vi "Create Files.vi"(8 "error in (no error)":errorcluster, 11 "CubeLogger in":refnum<class "CubeLogger.lvclass">) -> (0 "error out":errorcluster, 2 "Canceled?":bool, 3 "CubeLogger out":refnum<class "CubeLogger.lvclass">)   [LabVIEW 2018, in "CubeLogger.lvclass"]
uses:
  CubeLogger.lvclass
  CubeLogger.lvclass/CubeLogger.ctl
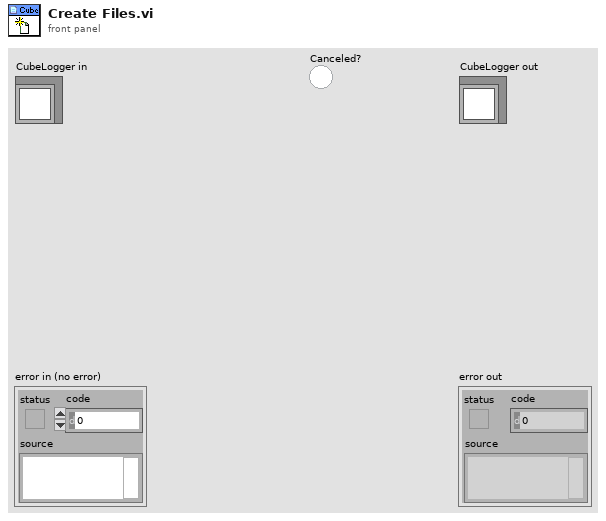
[diagram p1: front panel]
types:
  T1 = enum16{"open", "replace", "create", "open or create", "replace or create", "replace or create with confirmation"}
  T2 = typedef "CubeLogger.lvclass/Dataset.ctl" = cluster{"name":string, "path":string, "size":i32[], "type":enum16{"single", "double", "uint8", "uint16", "uint32", "uint64", "int8", "int16", "int32", "int64"}, "mfmt":string}
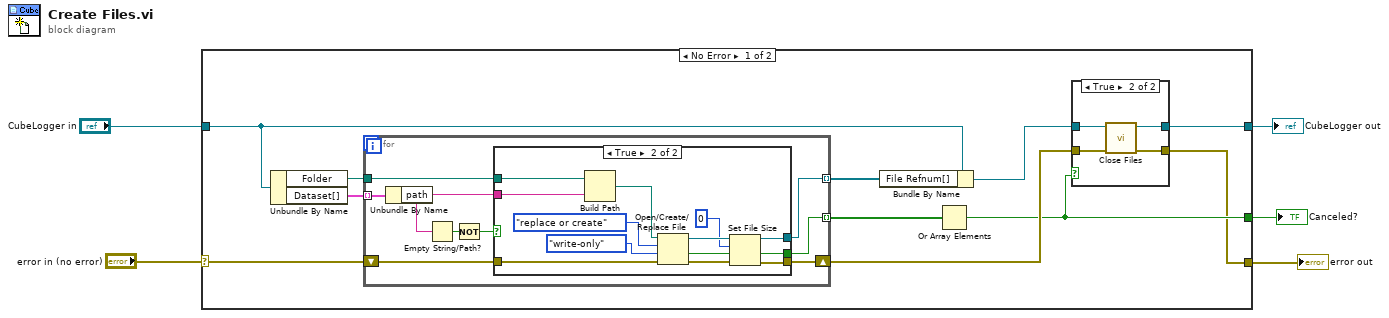
[diagram p0: block diagram]
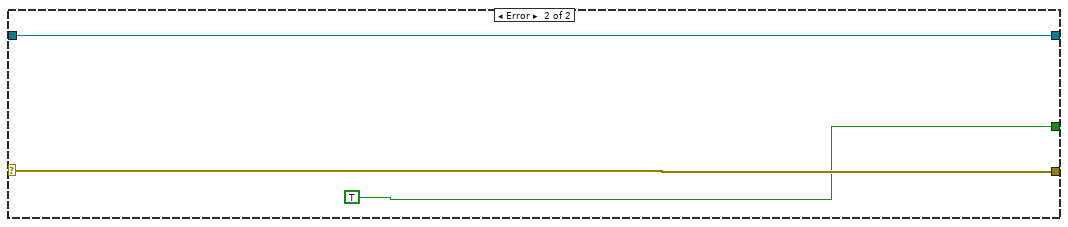
[diagram p4: hidden frame]
diagram:
  n1 = case shown="No Error" "error in (no error)" {
    selector: "error in (no error)" -> [w14 w47]
    tunnel: [w6 w47] -> w4
    tunnel: [w9 w46] -> w2
    tunnel: "CubeLogger in" -> [w12 w46]
    tunnel: [w7 TRUE] -> w1
    frame No Error {
      n2 = Unbundle By Name(w12) -> ("Folder"=w15:path, "Dataset[]"=w16:T2[])
      n3 = for {
        tunnel: w16 -> [w31] mode=indexing
        tunnel: w15 -> [w30]
        shift-right: [w28] -> w8
        shift-left: w14 -> [w29]
        tunnel: [w27] -> w13 mode=indexing
        tunnel: [w26] -> w11 mode=indexing
        n4 = Unbundle By Name(w31) -> ("path"=w24:string)
        n5 = Empty String/Path?(string/path=w24) -> (empty?=w25:bool)
        n6 = Not(x=w25) -> (.not. x?=w23:bool)
        n7 = case shown="True" w23 {
          tunnel: w24 -> [_ w44]
          tunnel: w30 -> [_ w43]
          tunnel: w29 -> [w32 w42]
          tunnel: [w32 w36] -> w28
          tunnel: [_ w41] -> w27
          tunnel: [_ w35] -> w26
          frame False {
          }
          frame True {
            n8 = Build Path(base path=w43, name or relative path=w44) -> (appended path=w40:path)
            n9 = Open/Create/Replace File(file path (use dialog)=w40, error in=w42, operation (0:open)=T1."replace or create", access (0:read/write)=enum16{"read/write", "read-only", "write-only"}."write-only") -> (refnum out=w34:refnum<file>, cancelled=w41:bool, error out=w37:errorcluster)  [unwired: 2 in]
            n10 = Set File Size(4:w37, 6:i64 0 ("size (in bytes)"), 7:w34) -> (0:w36:errorcluster, 3:w35:refnum<file>)
          }
        }
      }
      n11 = Bundle By Name(cluster=w12, "File Refnum[]"=w11) -> (w10:refnum<class "CubeLogger.lvclass">)
      n12 = Or Array Elements(Boolean array=w13) -> (logical OR=w7:bool)
      n13 = case shown="True" w7 {
        tunnel: w10 -> [w18 w22]
        tunnel: [w18 w21] -> w9
        tunnel: w8 -> [w17 w20]
        tunnel: [w17 w19] -> w6
        frame False {
        }
        frame True {
          n14 = call "Close Files.vi"("error in (no error)"=w20, "CubeLogger in"=w22) -> ("error out"=w19:errorcluster, "CubeLogger out"=w21:refnum<class "CubeLogger.lvclass">)  [unwired: 8 in]
        }
      }
    }
    frame Error {
    }
  }
  "error out" <- w4
  "CubeLogger out" <- w2
  "Canceled?" <- w1
